vi "GetSourceFormat.vi"(8 "Error In":errorcluster, 11 "Keithley 6482 In":refnum<visa-resource-name>) -> (0 "Error Out":errorcluster, 2 "Source Format":T1, 3 "Keithley 6482 Out":refnum<visa-resource-name>)   [LabVIEW 8.6, in "Keithley-6482-Visa.lvlib"]
uses:
  Keithley-6482-Visa.lvlib
  Controls/SourceFormat.ctl
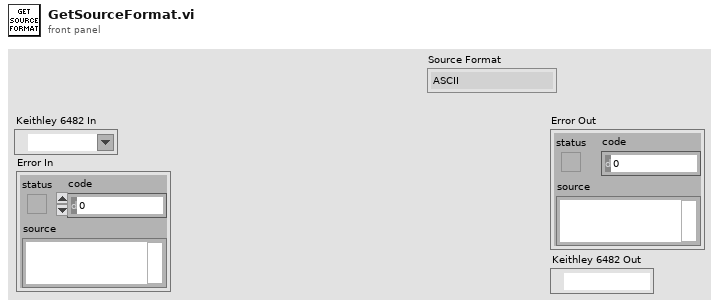
[diagram p1: front panel]
types:
  T1 = typedef "Keithley-6482-Visa.lvlib/SourceFormat.ctl" = enum16{"ASCII", "Hexadecimal", "Octal", "Binary"}
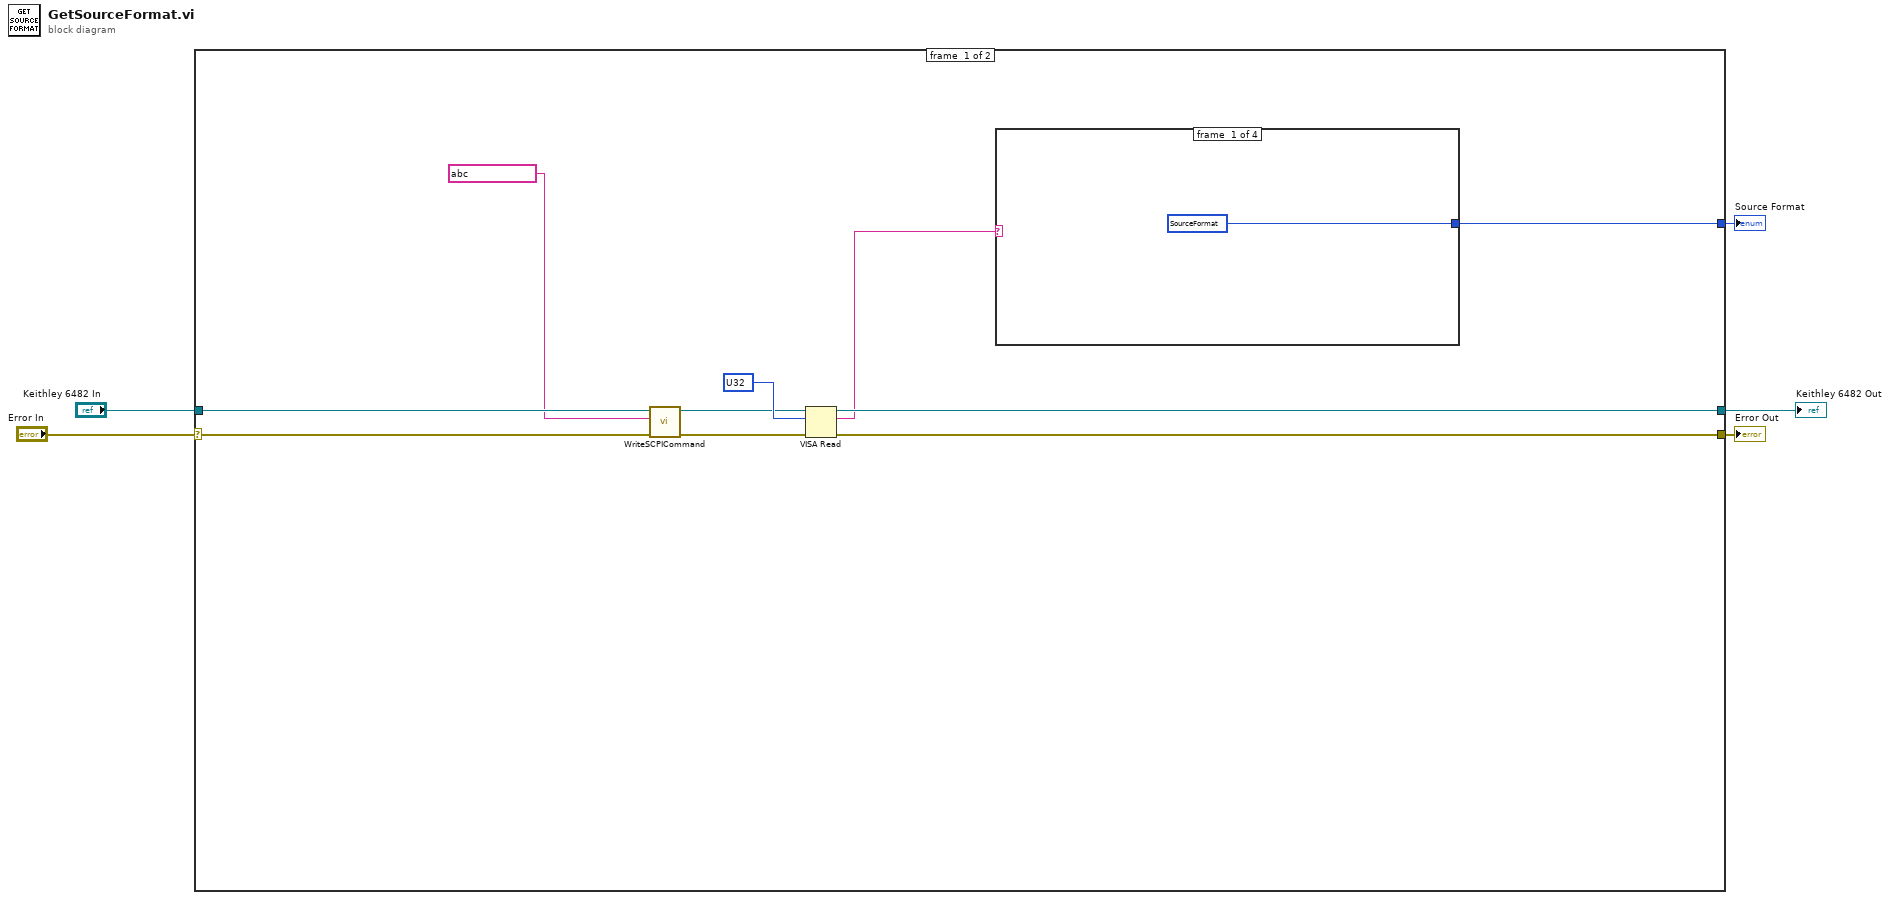
[diagram p0: block diagram]
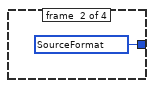
[diagram p2: hidden frame]
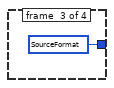
[diagram p3: hidden frame]
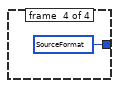
[diagram p4: hidden frame]
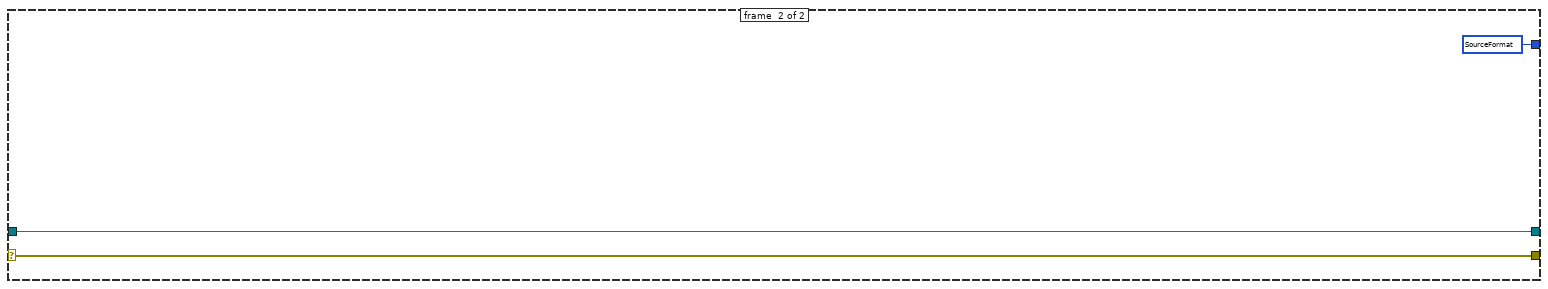
[diagram p5: hidden frame]
diagram:
  n1 = case shown="Error" "Error In" {
    selector: "Error In" -> [w10 w21]
    tunnel: "Keithley 6482 In" -> [w9 w22]
    tunnel: [w15 w21] -> w3
    tunnel: [w14 w22] -> w2
    tunnel: [w6 T1 ? ("Source Format")] -> w1
    frame #0 {
      n2 = call "WriteSCPICommand.vi"("Error In"=w10, "SCPI Command"=string ?, "Keithley 6482 In"=w9) -> ("Error Out"=w11:errorcluster, "Keithley 6482 Out"=w12:refnum<visa-resource-name>)  [unwired: 7 in]
      n3 = VISA Read(VISA resource name=w12, byte count=u32 ?, error in (no error)=w11) -> (VISA resource name out=w14:refnum<visa-resource-name>, read buffer=w7:string, error out=w15:errorcluster)  [unwired: 1 out]
      n4 = case shown="\"BIN\"" w7 {
        tunnel: [T1 ? ("Source Format") T1 ? ("Source Format") T1 ? ("Source Format") T1 ? ("Source Format")] -> w6
        frame #0 {
        }
        frame #1 {
        }
        frame #2 {
        }
        frame #3 {
        }
      }
    }
    frame #1 {
    }
  }
  "Error Out" <- w3
  "Keithley 6482 Out" <- w2
  "Source Format" <- w1
